vi "Store Configuration Parameters.vi"(8 "error in (no error)":errorcluster, 10 "refnum":T1, 11 "Example Configuration Dialog in":refnum<class "Example Configuration Dialog.lvclass">) -> (0 "error out":errorcluster, 2 "refnum out":T1, 3 "Example Configuration Dialog out":refnum<class "Example Configuration Dialog.lvclass">)   [LabVIEW 2017, in "Example Configuration Dialog.lvlib" / "Example Configuration Dialog.lvclass"]
uses:
  Example Configuration Dialog.lvclass
  <vilib>/Utility/config.llb/Config Data RefNum.ctl
  Example Configuration Dialog.lvclass/Example Configuration Dialog.ctl
  <vilib>/Utility/config.llb/Write Key (I32).vi
  <vilib>/Utility/config.llb/Write Key (String).vi
  Configuration.lvclass
  <vilib>/Utility/config.llb/NI_LVConfig.lvlib
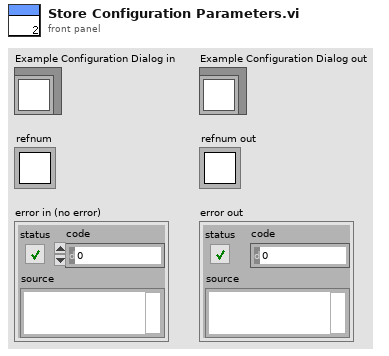
[diagram p1: front panel]
types:
  T1 = typedef "NI_LVConfig.lvlib/Config Data RefNum.ctl" = refnum<k1>
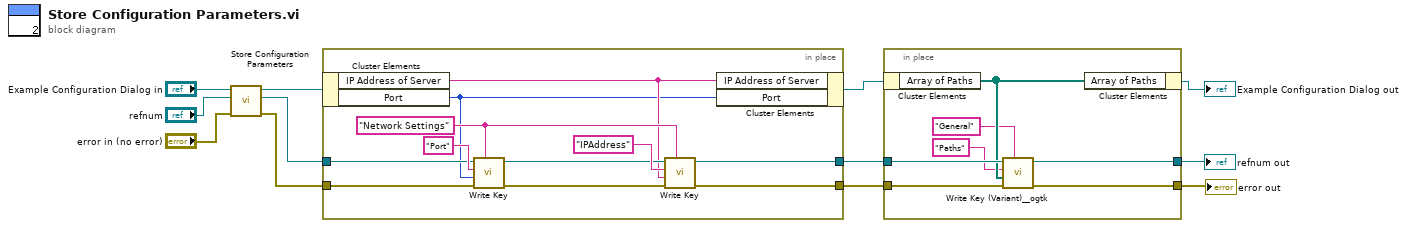
[diagram p0: block diagram]
diagram:
  n1 = call-parent "Store Configuration Parameters.vi"("error in (no error)"="error in (no error)", "refnum"="refnum", "Configuration in"="Example Configuration Dialog in") -> ("error out"=w8:errorcluster, "refnum out"=w9:T1, "Configuration out"=w7:refnum<class "Example Configuration Dialog.lvclass">)  [unwired: 6 in]
  n2 = in-place "In Place Element Structure" {
    in-place-border: w9 -> [w16]
    in-place-border: w8 -> [w20]
    in-place-border: [w22] -> w5
    in-place-border: [w21] -> w6
    w18 = "Network Settings" ("section")
    n3 = in-place-cluster #1(w7) -> ("IP Address of Server"=w14:string, "Port"=w13:i32)
    n4 = call-poly <vilib>:"Write Key.vi"("section"=w18, "error in (no error)"=w20, "value"=w13, "key"="Port", "refnum"=w16) -> ("error out"=w19:errorcluster, "refnum out"=w15:T1)  [unwired: 4 in, 1 out]
    n5 = call-poly <vilib>:"Write Key.vi"("section"=w18, "error in (no error)"=w19, "value"=w14, "key"="IPAddress", "refnum"=w15) -> ("error out"=w22:errorcluster, "refnum out"=w21:T1)  [unwired: 4 in, 1 out]
    n6 = in-place-cluster #1("IP Address of Server"=w14, "Port"=w13) -> (w4:refnum<class "Example Configuration Dialog.lvclass">)
  }
  n7 = in-place "In Place Element Structure" {
    in-place-border: w6 -> [w30]
    in-place-border: w5 -> [w29]
    in-place-border: [w25] -> w1
    in-place-border: [w24] -> w2
    n8 = in-place-cluster #2(w4) -> ("Array of Paths"=w28:path[])
    n9 = call <userlib>:"Write Key (Variant)__ogtk.vi"("section"="General", "error in (no error)"=w29, "key-value"=w28, "key (optional)"="Paths", "refnum"=w30) -> ("error out"=w25:errorcluster, "refnum out"=w24:T1)  [unwired: 5 in]
    n10 = in-place-cluster #2("Array of Paths"=w28) -> (→"Example Configuration Dialog out":refnum<class "Example Configuration Dialog.lvclass">)
  }
  "error out" <- w1
  "refnum out" <- w2
